vi "Add Control Caption.vi"(8 "error in (no error)":errorcluster, 11 "Tab in":refnum<class "Tab.lvclass">) -> (0 "error out":errorcluster, 3 "Tab out":refnum<class "Tab.lvclass">)   [LabVIEW 2017, in "Localization.lvlib" / "Tab.lvclass"]
doc: "VI for override that is supposed to do go throgh and create the Caption for the specific VI. Then the caption is set as visible and the label is hidden.\n\nChoose Movement Consulting, LLC"
uses:
  Tab.lvclass
  C:/Apps/CMC/OpenSource/Localization/Control Info/Control Info.lvclass
  Control Info/Control Info.lvclass
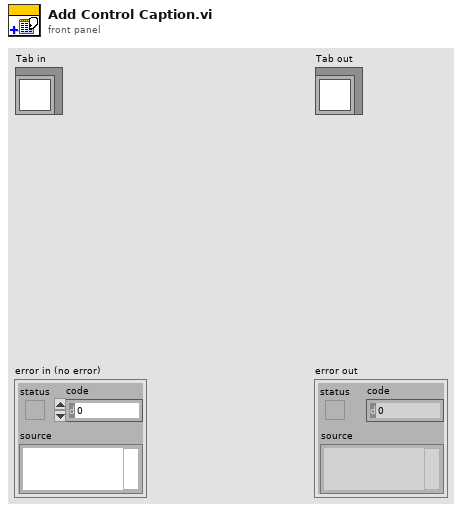
[diagram p1: front panel]
types:
  T1 = typedef "LVPositionTypeDef.ctl" = cluster{"Left":i32, "Top":i32}
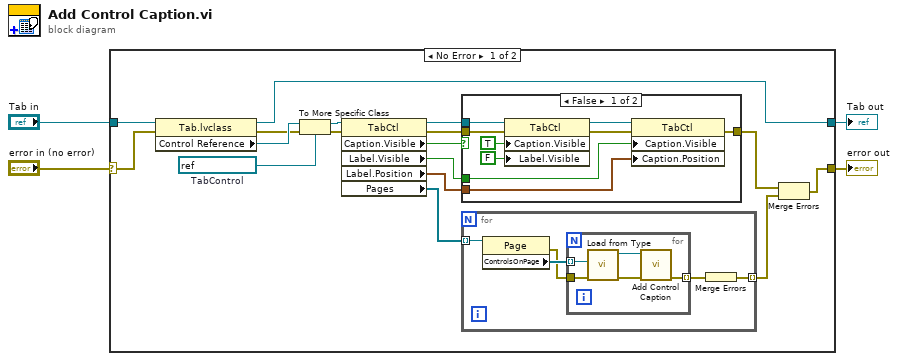
[diagram p0: block diagram]
diagram:
  n1 = case shown="No Error" "error in (no error)" {
    selector: "error in (no error)" -> [w16 w43]
    tunnel: "Tab in" -> [w15 w42]
    tunnel: [w12 w42] -> w1
    tunnel: [w9 w43] -> w2
    frame No Error {
      w17 = refnum<vi> refnum  # TabControl
      n2 = property class="Tab.lvclass"(reference=w15, error in=w16) -> (reference out=w12:refnum<class "Tab.lvclass">, error out=w20:errorcluster, "Control Reference"=w21:refnum<vi>)
      n3 = To More Specific Class(target class=w17, reference=w21, error in=w20) -> (specific class reference=w18:refnum<vi>, error out=w19:errorcluster)
      n4 = property class="TabCtl"(reference=w18, error in=w19) -> (reference out=w11:refnum<vi>, error out=w13:errorcluster, "Caption.Visible"=w14:bool, "Label.Visible"=w6:bool, "Label.Position"=w5:T1, "Pages"=w7:refnum<vi>[])
      n5 = case shown="False" w14 {
        tunnel: w13 -> [w39 w41]
        tunnel: w11 -> [w40 _]
        tunnel: [w34 w41] -> w10
        tunnel: w6 -> [w33 _]
        tunnel: w5 -> [w32 _]
        frame False {
          n6 = property class="TabCtl"(reference=w40, error in=w39, "Caption.Visible"=TRUE, "Label.Visible"=FALSE) -> (reference out=w36:refnum<vi>, error out=w35:errorcluster)
          n7 = property class="TabCtl"(reference=w36, error in=w35, "Caption.Visible"=w33, "Caption.Position"=w32) -> (error out=w34:errorcluster)  [unwired: 1 out]
        }
        frame True {
        }
      }
      n8 = for {
        tunnel: w7 -> [w26] mode=indexing
        tunnel: [w22] -> w8 mode=indexing
        n9 = property class="Page"(reference=w26) -> (error out=w24:errorcluster, "ControlsOnPage"=w25:refnum<vi>[])  [unwired: 1 in, 1 out]
        n10 = for {
          tunnel: w25 -> [w29] mode=indexing
          tunnel: w24 -> [w28]
          tunnel: [w27] -> w23 mode=indexing
          n11 = call "Load from Type.vi"("error in (no error)"=w28, "Control Reference"=w29) -> ("error out"=w31:errorcluster, "Control Info out"=w30:refnum<class "Control Info.lvclass">)  [unwired: 8 in]
          n12 = call-dynamic "Add Control Caption.vi"("error in (no error)"=w31, "Control Info in"=w30) -> ("error out"=w27:errorcluster)  [unwired: 8 in, 1 out]
        }
        n13 = Merge Errors(w23) -> (w22:errorcluster)
      }
      n14 = Merge Errors(w10, w8) -> (w9:errorcluster)
    }
    frame Error {
    }
  }
  "error out" <- w2
  "Tab out" <- w1
